vi "TH_CreateFilename.vi"() -> (0 "DataPath + Filename":path, 1 "DataPath":path, 2 "RootPath":path)   [LabVIEW 2014]
uses:
  TH_StartParameters.vi
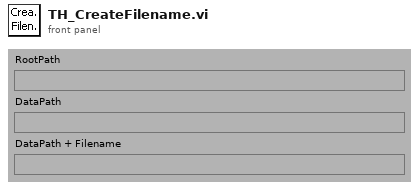
[diagram p1: front panel]
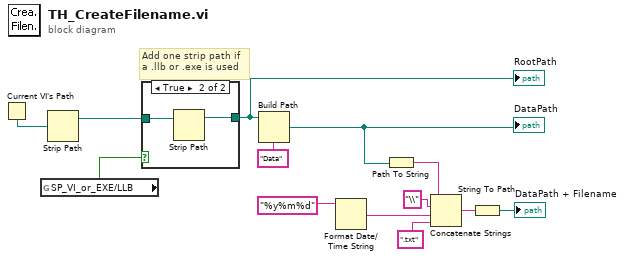
[diagram p0: block diagram]
diagram:
  # "Add one strip path if\na .llb or .exe is used"
  n1 = Current VI's Path() -> (path=w6:path)
  n2 = global read "TH_StartParameters.vi" "SP_VI_or_EXE/LLB"() -> (w3:bool)
  n3 = Strip Path(path=w6) -> (stripped path=w4:path)  [unwired: 1 out]
  n4 = case shown="True" w3 {
    tunnel: w4 -> [w14 w16]
    tunnel: [w14 w15] -> w1
    frame False {
    }
    frame True {
      n5 = Strip Path(path=w16) -> (stripped path=w15:path)  [unwired: 1 out]
    }
  }
  "RootPath" <- w1
  n6 = Build Path(base path=w1, name or relative path="Data") -> (appended path=w2:path)
  "DataPath" <- w2
  n7 = Format Date/Time String(time format string (%c)="%y%m%d") -> (date/time string=w10:string)  [unwired: 2 in]
  n8 = Path To String(path=w2) -> (string=w13:string)
  n9 = Concatenate Strings(w13, "\\" ("Substring"), w10, ".txt") -> (w12:string)
  n10 = String To Path(string=w12) -> (path=→"DataPath + Filename":path)
